vi "Get Hold Measurements.vi"(9 "Use Offsets":bool, 11 "LBCB Number":T2) -> (2 "Measurements":T1)   [LabVIEW 2009]
uses:
  Data Access Objects/Metadata/LBCB Number.ctl
  MixedMode/Mixed Mode Cartesian Data.ctl
  Cartesian Measurment Actions.ctl
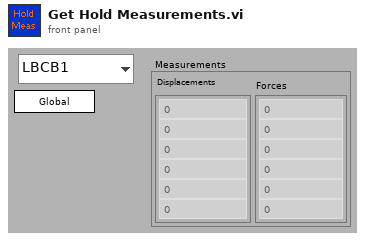
[diagram p1: front panel]
types:
  T1 = typedef "Mixed Mode Cartesian Data.ctl" = cluster{"Displacements":dbl[], "Forces":dbl[]}
  T2 = typedef "LBCB Number.ctl" = enum16{"LBCB1", "LBCB2"}
  T3 = typedef "Cartesian Measurment Actions.ctl" = enum16{"Set Data", "Get", "Init", "Set Offsets"}
  T4 = typedef "Cartesian Data Type.ctl" = cluster{"Displacements":dbl[], "Forces":dbl[], "Displacement Commands":dbl[]}
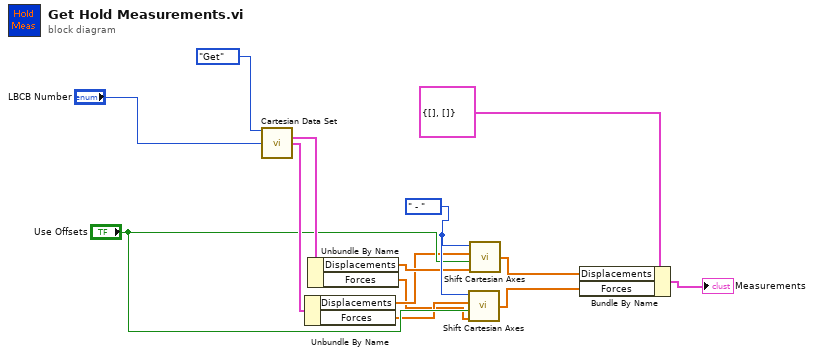
[diagram p0: block diagram]
diagram:
  w10 = enum16{" +", " - "}." - " ("Direction")
  n1 = call "Cartesian Data Set.vi"("Measurement Actions"=Cartesian_Measurment_Actions."Get", "LBCB Selected"="LBCB Number") -> ("Cartesian Data Offsets Out"=w11:T4, "Cartesian Data Hold Data Out"=w12:T4)  [unwired: 10 in, 2 out]
  n2 = Unbundle By Name(w12) -> ("Displacements"=w7:dbl[], "Forces"=w6:dbl[])
  n3 = Unbundle By Name(w11) -> ("Displacements"=w8:dbl[], "Forces"=w5:dbl[])
  n4 = call "Shift Cartesian Axes.vi"("Coordianate Offset"=w5, "Coordinate Switch"="Use Offsets", "Coordianate Input"=w6, "Direction"=w10) -> ("Coordianate Output"=w2:dbl[])
  n5 = call "Shift Cartesian Axes.vi"("Coordianate Offset"=w8, "Coordinate Switch"="Use Offsets", "Coordianate Input"=w7, "Direction"=w10) -> ("Coordianate Output"=w3:dbl[])
  n6 = Bundle By Name(cluster=T1 {"Displacements"=[], "Forces"=[]} ("Measurements"), "Displacements"=w3, "Forces"=w2) -> (→"Measurements":T1)
